vi "TopLevelFPGA.vi"() -> ()   [LabVIEW 2015]
uses:
  <vilib>/rvi/Emulation/niFpgaGetClockAttributes.vi
  <vilib>/rvi/Emulation/niFpgaSctlEmulationGetInTimedLoop.vi
  <vilib>/rvi/Emulation/niFpgaEmulationReportErrorSimple.vi
  <vilib>/rvi/eio/common/nirviEmuTemplateMethod_errors.vi
  <vilib>/rvi/Emulation/niFpgaCriticalErrorInLSC.vi
  <vilib>/eio/EIONode/EIONode.xnode
panel:
  in  "LED0_State":bool
  in  "WUC":bool=TRUE
  out "Duration 2":i16
  out "Count(mSec)":u32
  out "Button0":bool
  in  "DIO0_H":u32
  in  "DIO0_L":u32
  in  "LED3_H":u32
  in  "LED3_L":u32
  in  "LED2_H":u32
  in  "LED2_L":u32
  in  "LED1_L":u32
  in  "LED1_H":u32
  out "Acceleration":i16[](array[numeric])
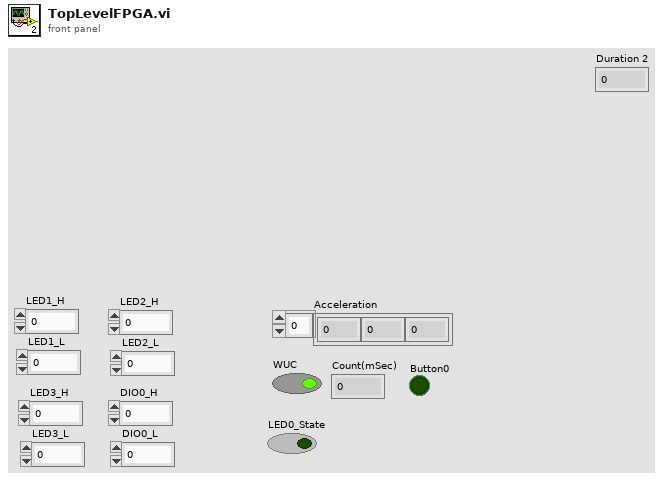
[diagram p1: front panel]
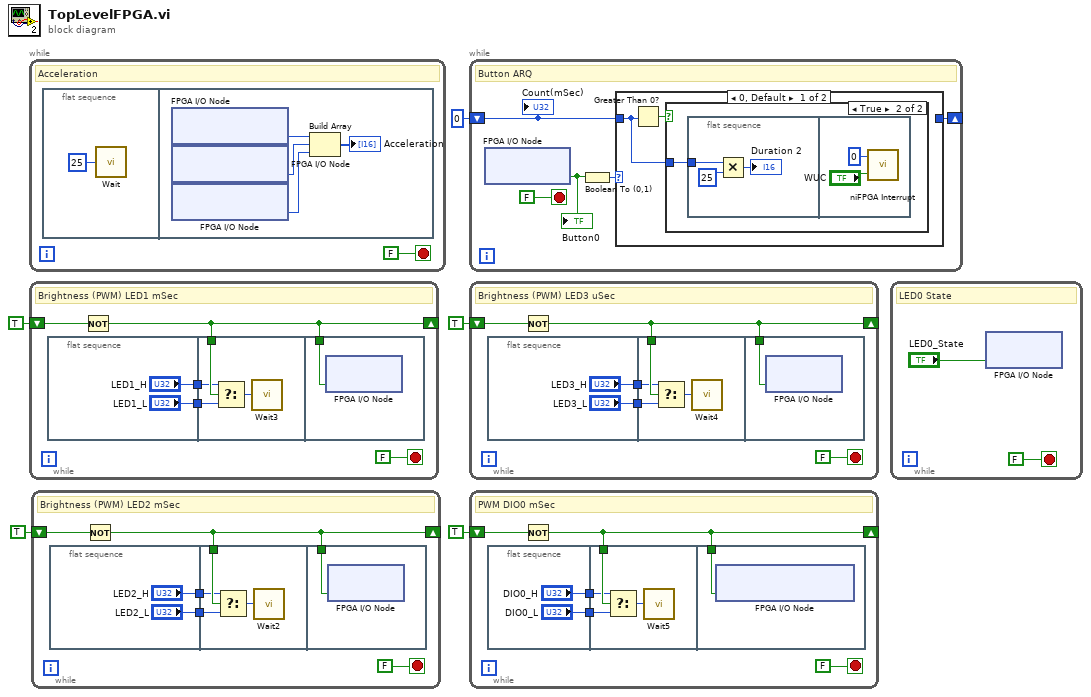
[diagram p0: block diagram]
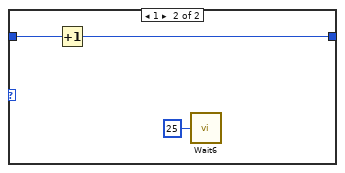
[diagram p3: hidden frame]
diagram:
  n1 = while {
    stop <- FALSE stop-if-true
    # "Acceleration"
    n2 = flat-sequence {
      frame #0 {
        n3 = call "Wait"("Count(mSec)"=u32 25) -> ()  [unwired: 1 out]
      }
      frame #1 {
        n4 = xnode "FPGA I/O Node"() -> ("AccelerationX"=w11:i16)  [unwired: 1 in, 1 out]
        n5 = xnode "FPGA I/O Node"() -> ("AccelerationY"=w10:i16)  [unwired: 1 in, 1 out]
        n6 = xnode "FPGA I/O Node"() -> ("AccelerationZ"=w9:i16)  [unwired: 1 in, 1 out]
        n7 = Build Array(w11, w10, w9) -> (→"Acceleration":i16[])
      }
    }
  }
  n8 = while {
    shift-right: [w13] -> _
    shift-left: TRUE -> [w14]
    stop <- FALSE stop-if-true
    # "Brightness (PWM) LED1 mSec"
    n9 = flat-sequence {
      tunnel: ["LED1_H"] -> w15
      tunnel: ["LED1_L"] -> w12
      tunnel: w15 -> [w20]
      tunnel: w13 -> [w21]
      tunnel: w12 -> [w19]
      tunnel: w13 -> [w23]
      frame #0 {
      }
      frame #1 {
        n10 = Select(t=w20, s=w21, f=w19) -> (s? t:f=w22:u32)
        n11 = call "Wait3"("Count(mSec)"=w22) -> ()  [unwired: 1 out]
      }
      frame #2 {
        n12 = xnode "FPGA I/O Node"("LED1"=w23) -> ()  [unwired: 1 in, 1 out]
      }
    }
    n13 = Not(x=w14) -> (.not. x?=w13:bool)
  }
  n14 = while {
    shift-right: [w25] -> _
    shift-left: TRUE -> [w26]
    stop <- FALSE stop-if-true
    # "Brightness (PWM) LED2 mSec"
    n15 = flat-sequence {
      tunnel: ["LED2_H"] -> w27
      tunnel: ["LED2_L"] -> w24
      tunnel: w27 -> [w32]
      tunnel: w25 -> [w33]
      tunnel: w24 -> [w31]
      tunnel: w25 -> [w35]
      frame #0 {
      }
      frame #1 {
        n16 = Select(t=w32, s=w33, f=w31) -> (s? t:f=w34:u32)
        n17 = call "Wait2"("Count(mSec)"=w34) -> ()  [unwired: 1 out]
      }
      frame #2 {
        n18 = xnode "FPGA I/O Node"("LED2"=w35) -> ()  [unwired: 1 in, 1 out]
      }
    }
    n19 = Not(x=w26) -> (.not. x?=w25:bool)
  }
  n20 = while {
    shift-right: [w37] -> _
    shift-left: u32 0 ("Count(mSec)") -> [w36]
    stop <- FALSE stop-if-true
    # "Button ARQ"
    n21 = xnode "FPGA I/O Node"() -> ("Button0"=w40:bool)  [unwired: 1 in, 1 out]
    "Button0" <- w40
    n22 = Boolean To (0,1)(Boolean=w40) -> (0, 1=w39:i16)
    n23 = case shown="0, Default" w39 {
      tunnel: [_ w49] -> w37
      tunnel: w36 -> [w41 w50]
      frame 0, Default {
        n24 = Greater Than 0?(x=w41) -> (x > 0?=w42:bool)
        n25 = case shown="True" w42 {
          tunnel: w41 -> [_ w43]
          frame False {
          }
          frame True {
            n26 = flat-sequence {
              tunnel: w43 -> [w44]
              frame #0 {
                n27 = Multiply(x=w44, y=i16 25) -> (x*y=→"Duration 2":u32)
              }
              frame #1 {
                n28 = call <vilib>:"niFPGA Interrupt.vi"("Wait Until Cleared (F)"="WUC", "IRQ Number (0)"=u8 0) -> ()  [unwired: 1 in]
              }
            }
          }
        }
      }
      frame 1 {
        n29 = Increment(x=w50) -> (x+1=w49:u32)
        n30 = call "Wait6"("Count(mSec)"=u32 25) -> ()  [unwired: 1 out]
      }
    }
    "Count(mSec)" <- w36
  }
  n31 = while {
    shift-right: [w53] -> _
    shift-left: TRUE -> [w54]
    stop <- FALSE stop-if-true
    # "Brightness (PWM) LED3 uSec"
    n32 = flat-sequence {
      tunnel: ["LED3_H"] -> w55
      tunnel: ["LED3_L"] -> w52
      tunnel: w55 -> [w60]
      tunnel: w53 -> [w61]
      tunnel: w52 -> [w59]
      tunnel: w53 -> [w63]
      frame #0 {
      }
      frame #1 {
        n33 = Select(t=w60, s=w61, f=w59) -> (s? t:f=w62:u32)
        n34 = call "Wait4"("Count(uSec)"=w62) -> ()  [unwired: 1 out]
      }
      frame #2 {
        n35 = xnode "FPGA I/O Node"("LED3"=w63) -> ()  [unwired: 1 in, 1 out]
      }
    }
    n36 = Not(x=w54) -> (.not. x?=w53:bool)
  }
  n37 = while {
    shift-right: [w65] -> _
    shift-left: TRUE -> [w66]
    stop <- FALSE stop-if-true
    # "PWM DIO0 mSec"
    n38 = flat-sequence {
      tunnel: ["DIO0_H"] -> w67
      tunnel: ["DIO0_L"] -> w64
      tunnel: w67 -> [w72]
      tunnel: w65 -> [w73]
      tunnel: w64 -> [w71]
      tunnel: w65 -> [w75]
      frame #0 {
      }
      frame #1 {
        n39 = Select(t=w72, s=w73, f=w71) -> (s? t:f=w74:u32)
        n40 = call "Wait5"("Count(mSec)"=w74) -> ()  [unwired: 1 out]
      }
      frame #2 {
        n41 = xnode "FPGA I/O Node"("ConnectorA/DIO0"=w75) -> ()  [unwired: 1 in, 1 out]
      }
    }
    n42 = Not(x=w66) -> (.not. x?=w65:bool)
  }
  n43 = while {
    stop <- FALSE stop-if-true
    # "LED0 State"
    n44 = xnode "FPGA I/O Node"("LED0"="LED0_State") -> ()  [unwired: 1 in, 1 out]
  }
